vi "input_torque.vi"(3 "error in (no error)":errorcluster, 4 "input":dbl, 5 "odrive":refnum<visa-resource-name>) -> (0 "error out":errorcluster, 2 "VISA resource name out":refnum<visa-resource-name>)   [LabVIEW 2019]
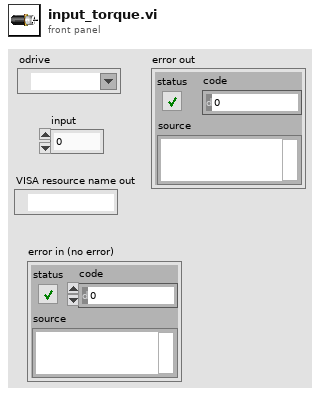
[diagram p1: front panel]
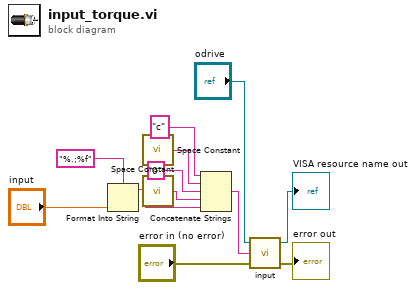
[diagram p0: block diagram]
diagram:
  n1 = Format Into String(format string="%.;%f", "input") -> (resulting string=w3:string)  [unwired: 2 in, 1 out]
  n2 = call <vilib>:"Space Constant.vi"() -> ("String"=w10:string)
  n3 = call <vilib>:"Space Constant.vi"() -> ("String"=w12:string)
  n4 = Concatenate Strings("c" ("write buffer"), w10, "0", w12, w3) -> (w8:string)
  n5 = call "input.vi"("error in (no error)"="error in (no error)", "commando"=w8, "VISA in"="odrive") -> ("error out"=→"error out":errorcluster, "VISA out"=→"VISA resource name out":refnum<visa-resource-name>)  [unwired: 1 out]
